vi "GEA2_CMD_WRITE_SETPOINTS.vi"(0 "ComPort":refnum<visa-resource-name>="COM1", 5 "Set Point":u8=140, 11 "Error In":errorcluster) -> (4 "ACK":bool, 15 "Error Out":errorcluster)   [LabVIEW 2014]
uses:
  Utility/GEA2 Commands/HEWH/Type Definitions/HEWH Command Type.ctl
  Utility/Labview GEA2 Toolkit v2.1/library/GEA2_Toolkit.lvlib
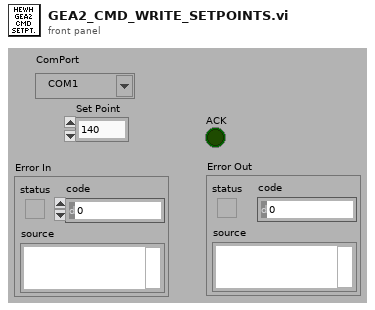
[diagram p1: front panel]
types:
  T1 = typedef "HEWH Command Type.ctl" = u8
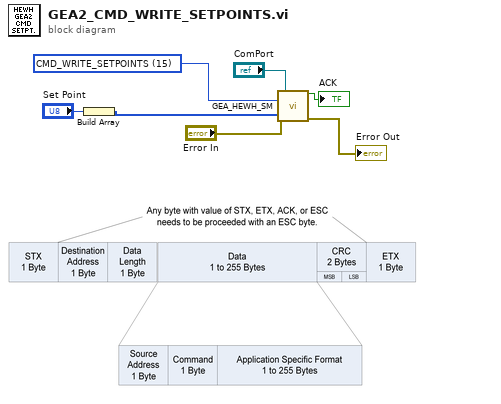
[diagram p0: block diagram]
diagram:
  w1 = T1 15 items=["RQST_SOFTWARE_VERSION", "RQST_T2_RESISTANCE", "RQST_T3A_RESISTANCE", "RQST_T3B_RESISTANCE", "RQST_T4_RESISTANCE", "RQST_T5_RESISTANCE", "RQST_IDLB_RESISTANCE", "RQST_MODE_SELECT_RESISTANCE", "RQST_DATA_FROM_MEMORY", "RQST_DATA_FROM_DATA_FLASH", "RQST_SS_FAULT_COUNTS", "RQST_OTHER_FAULT_COUNTS", "CMD_CLEAR_FAULT_COUNTS", "RQST_HYPERTERM_OUTPUT_DATA", "CMD_RESET_FILTER_TIMES", "CMD_WRITE_SETPOINTS", "CMD_TURN_ON_OFF_DLB", "CMD_ENTER_EXIT_FCT_MODE", "CMD_SET_LEDS", "CMD_SET_EEV_DRIVE_LINES", "REQ_READ_KEY_STATUS", "RQST_READ_PERSONALITY", "CMD_ENTER_FACT_MODE", "CMD_RESET", "CMD_RESTORE_EEPROM_DEFAULTS", "CMD_SET_MODEL_NUMBER", "CMD_SET_SERIAL_NUMBER", "RQST_MODEL_NUMBER", "RQST_SERIAL_NUMBER", "CMD_TOGGLE_SERVICE_MODE", "CMD_TOGGLE_UE_SERV", "CMD_TOGGLE_LE_SERV", "CMD_REFRESH_SERVICE_TIMEOUTS", "RQST_DSM_OVERRIDE_STATUS", "RQST_STATUS_QUERY", "RQST_HEM_KWH_DATA", "RQST_SERVICE_ERROR_CODES", "RQST_OVERRIDE_STATUS", "CMD_UPDATE_DSM_LEVEL", "CMD_OVERRIDE_STATUS_CHANGED", "CMD_CLEAR_OVERRIDE_STATUS", "CMD_CLEAR_ENERGY_USAGE_CTRS", "CMD_DSM_OVERRIDES", "CMD_UPDATE_MODE", "CMD_SET_PID_P_DENOMINATOR", "CMD_SET_PID_I_DENOM_UNDER_THR", "CMD_SET_PID_I_DENOM_OVER_THR", "CMD_SET_START_POS_UNDER_THR", "CMD_SET_START_POS_OVER_THR", "CMD_SET_EEV_STOP_POSITION", "CMD_SET_AMBIENT_THRESH_1", "CMD_SET_AMBIENT_THRESH_2", "CMD_SET_AMBIENT_THRESH_3", "CMD_SET_PID_LOW_SH_TARGET", "CMD_SET_PID_MID_SH_TARGET", "RQST_PID_PARAMETERS", "CMD_COMP_OFF", "CMD_TOGGLE_FAN", "CMD_RQST_LED_STATUS", "CMD_UE_2_SECONDS", "CMD_LE_2_SECONDS", "CMD_COMP_ON", "CMD_HP_RUN_6MIN", "RQST_TEMP_RANGE", "RQST_VACATION_RANGE", "RQST_STD_ELEC_RANGE", "RQST_WATER_CAPACITY", "CMD_CANCEL_EEV_POSITION", "CMD_EEV_POSITION", "CMD_SET_CURRENTS", "RQST_SUPPORTED_MODES"] ("Command")
  n1 = Build Array("Set Point") -> (w4:u8[])
  n2 = call "GEA_HEWH_SM.vi"("ComPort"="ComPort", "Command"=w1, "Command Data"=w4, "Error In"="Error In") -> ("WriteACK"=→"ACK":bool, "Error Out"=→"Error Out":errorcluster)  [unwired: 7 in, 3 out]
